vi "Class - Inheritance.vi"(7 "Msg Chain":string, 8 "error in (no error)":errorcluster {"code" format="Error %.0f"}, 10 "Classes":refnum<class "Class Documentation.lvclass">[](array[class]), 11 "VIDoc Printer - Confluence In":refnum<class "VIDoc Printer - Confluence.lvclass">) -> (0 "error out":errorcluster {"code" format="Error %.0f"}, 3 "VIDoc Printer - Confluence Out":refnum<class "VIDoc Printer - Confluence.lvclass">)   [LabVIEW 2023, in "VIDoc Printer - Confluence.lvlib" / "VIDoc Printer - Confluence.lvclass"]
uses:
  VIDoc Printer - Confluence.lvclass
  C:/projects/DMC/Tooling/Git-Action-Service/Source/Documentation Generation/Printers/Printer/VIDoc Printer.lvclass
  Parsing/Class Documentation/Class Documentation.lvclass
  Parsing/Class Documentation/Class Documentation.lvclass/Class Documentation.ctl
  Confluence Formatting/Types/Format Combo Box.ctl
  Parsing/Class Documentation/Get Parent Classes.vi
  Parsing/Class Documentation/Get Parent Interfaces.vi
  Parsing/Class Documentation/Get Parent Libraries.vi
  Parsing/Class Documentation/Get Class_Library.vi
  Parsing/Class Documentation/Get Name.vi
  VIDoc Printer - Confluence.lvclass/VIDoc Printer - Confluence.ctl
  Printer/VIDoc Printer.lvclass
  UI Interaction/UI Interaction.lvclass
  Confluence Formatting/Confluence Formatting.lvlib
  C:/projects/DMC/Tooling/Git-Action-Service/Source/Documentation Generation/Printers/Confluence Printer/VIDoc Printer - Confluence.lvclass
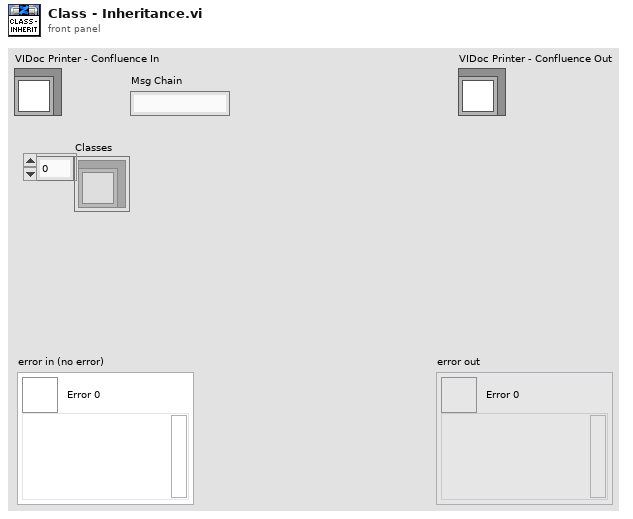
[diagram p1: front panel]
types:
  T1 = typedef "Confluence Formatting.lvlib/Format Combo Box.ctl" = string
  T2 = typedef "VIDoc Parsing.lvlib/Base Class Info Cluster.ctl" = cluster{"Name":string, "Icon":T3, "Version":cluster{"Major":u16, "Minor":u16, "Fix":u16, "Build":u16}, "Description":string, "Friends":string[], "ChildRefsRestricted":bool, "TransferMustOverrides":bool, "Path":path, "Qualified Name":string, "Class Scope":enum32{"invalid scope", "public", "private", "protected", "community"}}
  T3 = typedef "imagedata.ctl" = cluster{"image type":i32, "image depth":i32, "image":u8[], "mask":u8[], "colors":u32[], "Rectangle":cluster{"left":i16, "top":i16, "right":i16, "bottom":i16}}
  T4 = typedef "NI.Parent Library Information.ctl" = cluster{"qualified name":string, "localized name":string, "path":path, "parent library kind":T5}
  T5 = typedef "NI.Parent Library Kind.ctl" = enum32{"unknown", "class", "interface"}
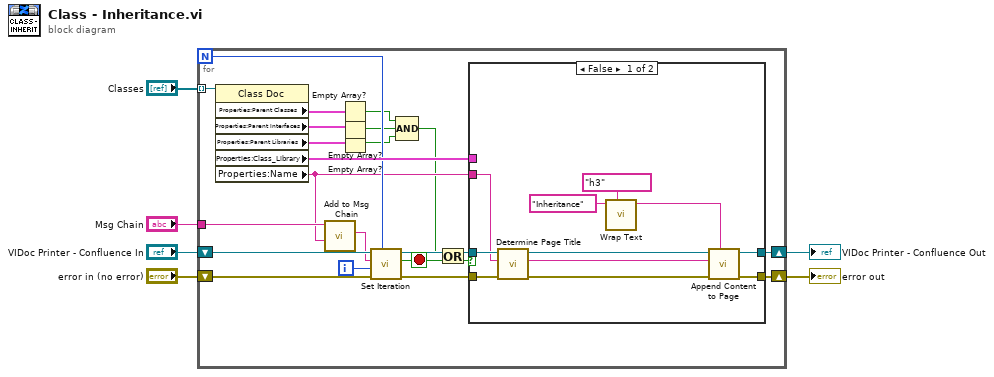
[diagram p0: block diagram]
diagram:
  n1 = for {
    N -> [w20]
    shift-right: [w26] -> w2
    shift-left: "error in (no error)" -> [w23]
    shift-right: [w27] -> w1
    shift-left: "VIDoc Printer - Confluence In" -> [w24]
    tunnel: "Classes" -> [w28] mode=indexing
    tunnel: "Msg Chain" -> [w18]
    i -> [w19]
    stop <- w15 stop-if-true
    n2 = property class="Class Doc"(reference=w28) -> ("Properties:Parent Classes"=w14:T2[], "Properties:Parent Interfaces"=w13:T2[], "Properties:Parent Libraries"=w12:T4[], "Properties:Class_Library"=w25:T2, "Properties:Name"=w17:string)  [unwired: 1 in, 2 out]
    n3 = call "Add to Msg Chain.vi"("New"=w17, "Msg Chain in"=w18) -> ("Msg Chain out"=w16:string)  [unwired: 9 in]
    n4 = Empty Array?(array=w14) -> (empty?=w10:bool)
    n5 = Empty Array?(array=w13) -> (empty?=w11:bool)
    n6 = Empty Array?(array=w12) -> (empty?=w9:bool)
    n7 = call "Set Iteration.vi"("Progress Max"=w20, "error in (no error)"=w23, "Progress Value"=w19, "Message (No Message Update)"=w16, "VIDoc Printer In"=w24) -> ("error out"=w21:errorcluster, "Abort?"=w15:bool, "VIDoc Printer Out"=w22:refnum<class "VIDoc Printer - Confluence.lvclass">)  [unwired: 4 in]
    n8 = Compound Arithmetic op=AND(w10, w11, w9) -> (w7:bool)
    n9 = Or(x=w7, y=w15) -> (x .or. y?=w8:bool)
    n10 = case shown="False" w8 {
      tunnel: [w36 w40] -> w27
      tunnel: [w35 w41] -> w26
      tunnel: w25 -> [_ _]
      tunnel: w22 -> [w33 w40]
      tunnel: w21 -> [w32 w41]
      tunnel: w17 -> [w31 _]
      frame False {
        n11 = call "Determine Page Title.vi"("error in (no error)"=w32, "Name"=w31, "VIDoc Printer - Confluence In"=w33) -> ("error out"=w38:errorcluster, "Page Title"=w39:string, "VIDoc Printer - Confluence Out"=w37:refnum<class "VIDoc Printer - Confluence.lvclass">)  [unwired: 5 in, 1 out]
        n12 = call "Wrap Text.vi"("Formatting"=T1 "h3", "String"="Inheritance") -> ("Wrapped String"=w29:string)  [unwired: 8 in, 1 out]
        n13 = call "Append Content to Page.vi"("Page Content"=w29, "error in (no error)"=w38, "Page Title"=w39, "VIDoc Printer - Confluence In"=w37) -> ("error out"=w35:errorcluster, "VIDoc Printer - Confluence Out"=w36:refnum<class "VIDoc Printer - Confluence.lvclass">)  [unwired: 6 in]
      }
      frame True {
      }
    }
  }
  "error out" <- w2
  "VIDoc Printer - Confluence Out" <- w1
